vi "ECUSignalSender_Create.vi"() -> (14 "EventHandl(订阅事件用)":refnum<event-registration>[](array[refnum]), 15 "SMOArry":refnum<class "SignalSenderLoop.lvclass">[](array[class]), 19 "错误输出":errorcluster)   [LabVIEW 2020]
uses:
  Typedefs/PublicEvents--Cluster.ctl
  Typedefs/SetpointChanged--EventData--Cluster.ctl
  Typedefs/Data.ctl
  <vilib>/JKI/JKI SMO/SMO/Typedefs/Public Events.ctl
  <vilib>/JKI/JKI SMO/SMO/Typedefs/SMOState --Enum.ctl
  <vilib>/JKI/JKI SMO/SMO/Typedefs/Reserve State--Enum.ctl
  SignalSenderLoop.lvclass
  C:/Program Files (x86)/National Instruments/LabVIEW 2020/vi.lib/JKI/JKI SMO/SMO/SMO.lvclass
  <vilib>/JKI/JKI SMO/SMO/SMO.lvclass/SMO.ctl
  <vilib>/JKI/JKI SMO/SMO/Private/ReftoDVR--SMO.vi
  <vilib>/JKI/JKI SMO/SMO/SMO.lvclass
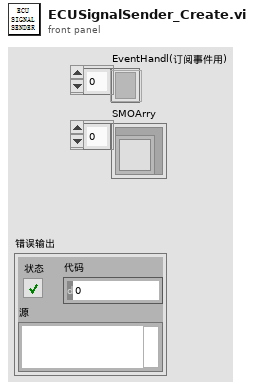
[diagram p1: front panel]
types:
  T1 = typedef "ECU_Diagnose.lvlib/SignalSenderLoop.lvclass/SignalFrameSet.ctl" = cluster{"Port_No.":refnum<k21>, "计数Count":bool, "校验CheckSum":bool, "MessageFrame":refnum<k21>, "校验算法名称":string}
  T2 = typedef "SMO.lvclass/Public Events.ctl" = cluster{"Error":refnum<user-event>, "State":refnum<user-event>, "Reserve State":refnum<user-event>}
  T3 = typedef "ECU_Diagnose.lvlib/SignalSenderLoop.lvclass/PublicEvents--Cluster.ctl" = cluster{"Setpoint Changed":refnum<user-event>, "Value Changed":refnum<user-event>}
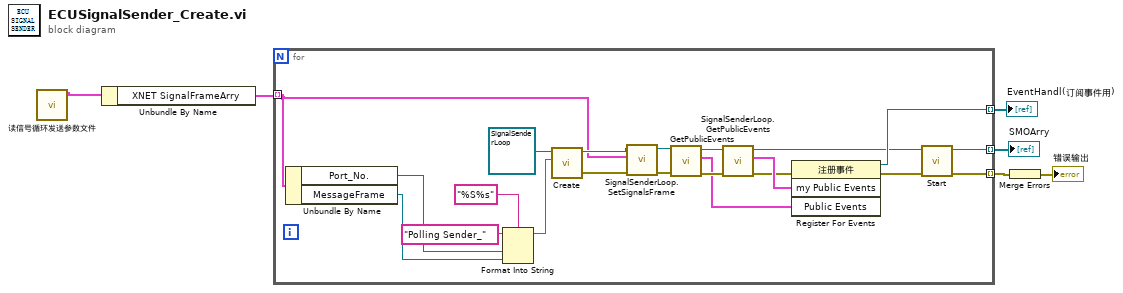
[diagram p0: block diagram]
diagram:
  n1 = call "读信号循环发送参数文件.vi"() -> ("信号轮询发送设置Out"=w1:cluster{"XNET SignalFrameArry":T1[]})  [unwired: 18 in, 1 out]
  n2 = Unbundle By Name(w1) -> ("XNET SignalFrameArry"=w6:T1[])
  n3 = for {
    tunnel: w6 -> [w9] mode=indexing
    tunnel: [w14] -> w5 mode=indexing
    tunnel: [w11] -> w4 mode=indexing
    tunnel: [w10] -> w3 mode=indexing
    n4 = Unbundle By Name(w9) -> ("Port_No."=w8:refnum<k21>, "MessageFrame"=w7:refnum<k21>)
    n5 = Format Into String(format string="%S%s" ("格式字符串"), initial string="Polling Sender_", w8, w7) -> (resulting string=w15:string)  [unwired: 1 in, 1 out]
    n6 = call <vilib>:"Create.vi"("Subsystem Name (optional)"=w15, "SMO"=refnum<class "SignalSenderLoop.lvclass"> refnum ("SMO.Template.lvclass")) -> ("error out"=w17:errorcluster, "SMO out"=w19:refnum<class "SignalSenderLoop.lvclass">)  [unwired: 7 in, 1 out]
    n7 = call "SignalSenderLoop.SetSignalsFrame.vi"("error in (no error)"=w17, "SignalFrameSet"=w9, "SignalSenderLoop"=w19) -> ("error out"=w16:errorcluster, "SignalSenderLoop out"=w18:refnum<class "SignalSenderLoop.lvclass">)  [unwired: 7 in]
    n8 = call <vilib>:"GetPublicEvents.vi"("error in (no error)"=w16, "SMO"=w18) -> ("error out"=w23:errorcluster, "Public Events"=w20:T2, "SMO out"=w22:refnum<class "SignalSenderLoop.lvclass">)  [unwired: 7 in]
    n9 = call "SignalSenderLoop.GetPublicEvents.vi"("error in (no error)"=w23, "SignalSenderLoop"=w22) -> ("error out"=w21:errorcluster, "my Public Events"=w24:T3, "SignalSenderLoop out"=w13:refnum<class "SignalSenderLoop.lvclass">)  [unwired: 7 in]
    n10 = register-events(error in=w21, w24, w20) -> (reference out=w14:refnum<event-registration>, error out=w12:errorcluster)  [unwired: 1 in]
    n11 = call <vilib>:"Start.vi"("error in (no error)"=w12, "SMO"=w13) -> ("error out"=w10:errorcluster, "SMO out"=w11:refnum<class "SignalSenderLoop.lvclass">)  [unwired: 8 in]
  }
  "EventHandl(订阅事件用)" <- w5
  "SMOArry" <- w4
  n12 = Merge Errors(w3) -> (→"错误输出":errorcluster)
